vi "Element Hierarchy.vi"(7 "Elements":refnum<class "Config Element.lvclass">[](array[class]), 8 "error in (no error)":errorcluster, 10 "Config Element in":refnum<class "Config Element.lvclass">) -> (0 "error out":errorcluster, 2 "Hierarchy":string[](array[string]))   [LabVIEW 2020, in "CDM-Config.lvlib" / "Config Manager.lvclass"]
doc: "This is a Manager internal VI for getting element hierarchy meant to be used within an IPE of the manager reference. The Config Element.lvclass' hierarchy VI required calling back into the manager to retrieve parents which would deadlock when called from within an already unlocked manager ref."
uses:
  Config Manager.lvclass
  Config Manager.lvclass/Config Manager.ctl
  Config Element/Config Element.lvclass
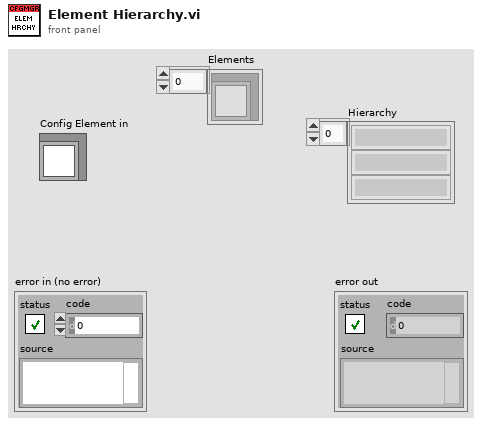
[diagram p1: front panel]
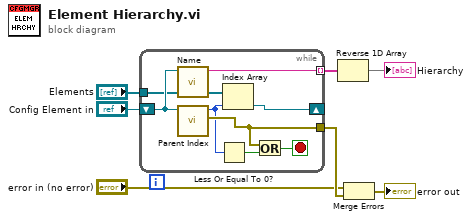
[diagram p0: block diagram]
diagram:
  n1 = while {
    shift-right: [w10] -> _
    shift-left: "Config Element in" -> [w12]
    tunnel: [w15] -> w7 mode=indexing
    tunnel: [w9] -> w3
    tunnel: "Elements" -> [w11]
    stop <- w13 stop-if-true
    n2 = call "Name.vi"("Config Element in"=w12) -> ("Name"=w15:string)  [unwired: 9 in, 1 out]
    n3 = call "Parent Index.vi"("Config Element in"=w12) -> ("error out"=w9:errorcluster, "Parent Index"=w8:i32)  [unwired: 9 in]
    n4 = Less Or Equal To 0?(x=w8) -> (x <= 0?=w14:bool)
    n5 = Index Array(array=w11, index=w8) -> (element=w10:refnum<class "Config Element.lvclass">)
    n6 = Or(x=w9, y=w14) -> (x .or. y?=w13:bool)
  }
  n7 = Reverse 1D Array(array=w7) -> (reversed array=→"Hierarchy":string[])
  n8 = Merge Errors("error in (no error)", w3) -> (→"error out":errorcluster)
